vi "Get 2D Array Double.vi"(5 "use temporary file? (F)":bool, 7 "data type of variable":dbl[][](array[numeric]), 8 "error in":errorcluster, 10 "variable name":string, 11 "GOLPI ref. in":T1={"pipe handle"={"lv_proc.dll file path"=path "", "process instance handle"=[], "debug mode"=FALSE, "debug data"=[]}, "fast read timeout [ms]"=500, "fast read settle time [ms]"=10, "fast read to multiple [ms]"=1, "max elements per input line"=100, "slow read timeout [ms]"=5000, "stdin double format specifier"="%_16e", "max elements per stdout output column"=100}) -> (0 "error out":errorcluster, 2 "value":dbl[][](array[numeric]) format="%.2f", 3 "GOLPI ref. out":T1={"pipe handle"={"lv_proc.dll file path"=path "", "process instance handle"=[], "debug mode"=FALSE, "debug data"=[]}, "fast read timeout [ms]"=500, "fast read settle time [ms]"=10, "fast read to multiple [ms]"=1, "max elements per input line"=100, "slow read timeout [ms]"=5000, "stdin double format specifier"="%_16e", "max elements per stdout output column"=100})   [LabVIEW 2013, in "GOLPI library.lvlib"]
doc: "Part of polymorph Get Variable.vi"
uses:
  GOLPI library.lvlib
  Public/GOLPI reference Type Def.ctl
  LV Process source distribution/Pipe Handle.ctl
  Type Definitions/Custom Error Codes Enum Type Def.vi
  LV Process source distribution/LV Process library.lvlib
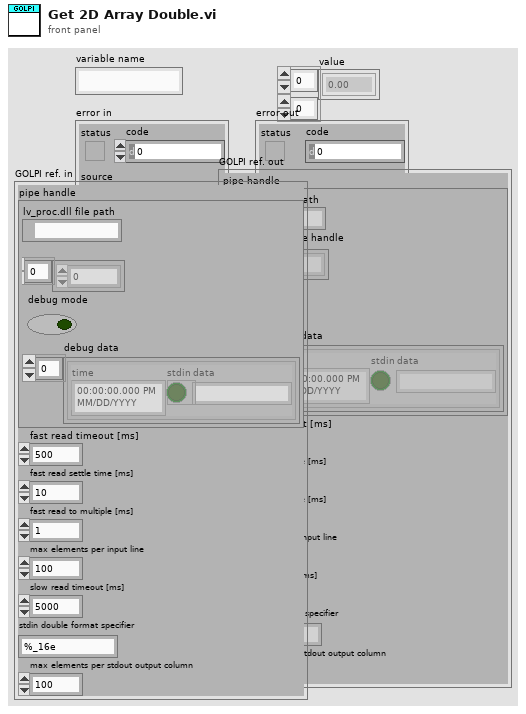
[diagram p1: front panel]
types:
  T1 = typedef "GOLPI library.lvlib/GOLPI reference Type Def.ctl" = cluster{"pipe handle":T2, "fast read timeout [ms]":u32, "fast read settle time [ms]":u32, "fast read to multiple [ms]":u32, "max elements per input line":u32, "slow read timeout [ms]":u32, "stdin double format specifier":string, "max elements per stdout output column":u32}
  T2 = typedef "LV Process library.lvlib/Pipe Handle.ctl" = cluster{"lv_proc.dll file path":path, "process instance handle":u32[], "debug mode":bool, "debug data":cluster{"time":timestamp, "stdin":bool, "data":string}[]}
  T3 = typedef "GOLPI library.lvlib/Custom Error Codes Enum Type Def.vi" = enum16{"no error", "00 working directory PAR1 missing", "01 octave binary PAR1 missing", "02 octave report error PAR1", "03 empty output last cmd PAR1", "04 missing temporary file PAR1", "05 pwd PAR 1 not exist", "10 var PAR1 not string, vect", "11 var PAR1 not num, scal, ~compl", "12 var PAR1 not num, scal, compl", "13 var PAR1 not num, vect, ~compl", "14 var PAR1 not num, vect, compl", "15 var PAR1 not num, mat, ~compl", "16 var PAR1 not num, mat, ~compl", "30 WARNING read timeout", "99 not finished"}
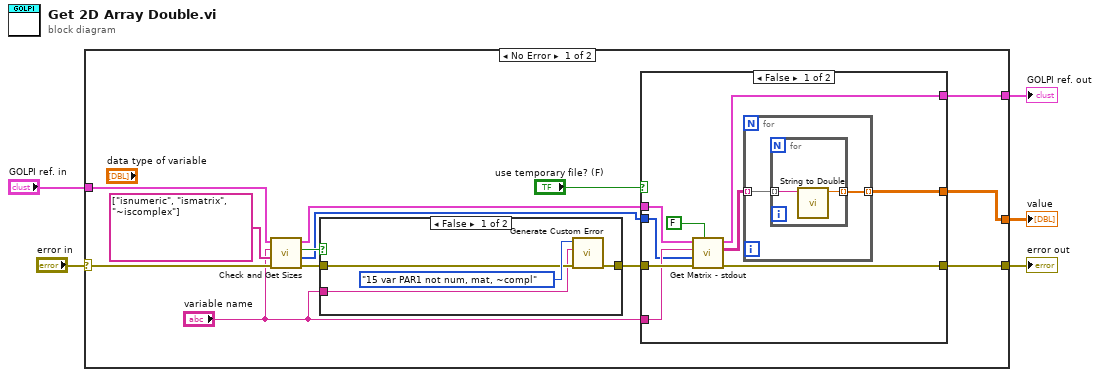
[diagram p0: block diagram]
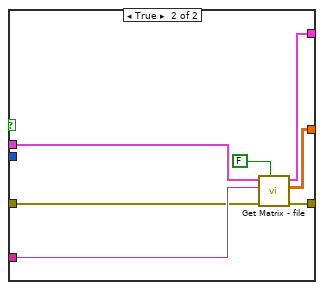
[diagram p2: hidden frame]
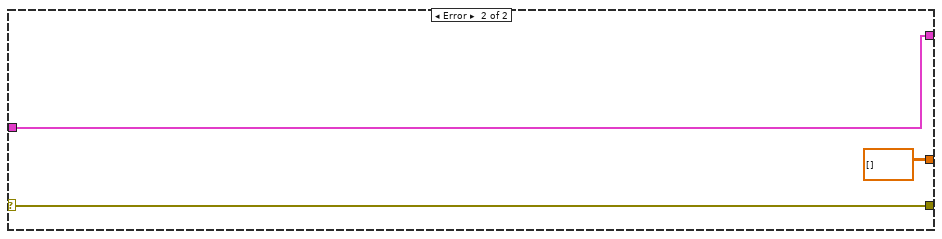
[diagram p4: hidden frame]
diagram:
  n1 = case shown="No Error" "error in" {
    selector: "error in" -> [w16 w46]
    tunnel: [w11 w46] -> w5
    tunnel: [w18 dbl[][] [] ("double array")] -> w3
    tunnel: "GOLPI ref. in" -> [w8 w44]
    tunnel: [w7 w44] -> w1
    frame No Error {
      n2 = call "Check and Get Sizes.vi"("error in (no error)"=w16, "test commands"=string[] ["isnumeric", "ismatrix", "~iscomplex"], "variable name"="variable name", "GOLPI ref. in"=w8) -> ("error out"=w15:errorcluster, "octave sizes"=w6:i32[], "all tests OK?"=w17:bool, "GOLPI ref. out"=w13:T1)  [unwired: 4 in]
      n3 = case shown="False" w17 {
        tunnel: w15 -> [w41 w43]
        tunnel: [w40 w43] -> w12
        tunnel: "variable name" -> [w39 _]
        frame False {
          n4 = call "Generate Custom Error.vi"("error in"=w41, "PAR1"=w39, "GOLPI error"=Custom_Error_Codes_Enum_Type_Def.vi."15 var PAR1 not num, mat, ~compl" ("Enum")) -> ("error out"=w40:errorcluster)  [unwired: 8 in]
        }
        frame True {
        }
      }
      n5 = case shown="False" "use temporary file? (F)" {
        tunnel: [w19 w32] -> w18
        tunnel: w13 -> [w24 w37]
        tunnel: [w21 w36] -> w7
        tunnel: w12 -> [w27 w34]
        tunnel: [w26 w33] -> w11
        tunnel: "variable name" -> [w25 w35]
        tunnel: w6 -> [w22 _]
        frame False {
          n6 = call "Get Matrix - stdout.vi"("is string?"=FALSE ("is string"), "error in (no error)"=w27, "octave sizes"=w22, "variable name"=w25, "GOLPI ref. in"=w24) -> ("error out"=w26:errorcluster, "array"=w20:string[][], "GOLPI ref. out"=w21:T1)  [unwired: 4 in]
          n7 = for {
            tunnel: w20 -> [w29] mode=indexing
            tunnel: [w28] -> w19 mode=indexing
            n8 = for {
              tunnel: w29 -> [w31] mode=indexing
              tunnel: [w30] -> w28 mode=indexing
              n9 = call "String to Double.vi"("string"=w31) -> ("number"=w30:dbl)  [unwired: 10 in]
            }
          }
        }
        frame True {
          n10 = call "Get Matrix - file.vi"("is string?"=FALSE ("is string"), "error in (no error)"=w34, "variable name"=w35, "GOLPI ref. in"=w37) -> ("error out"=w33:errorcluster, "double array"=w32:dbl[][], "GOLPI ref. out"=w36:T1)  [unwired: 3 in, 2 out]
        }
      }
    }
    frame Error {
    }
  }
  "value" <- w3
  "error out" <- w5
  "GOLPI ref. out" <- w1
